vi "Check Protection.vi"(8 "error in (no error)":errorcluster, 10 "String in":string, 11 "SMC Protection in":refnum<class "SMC Protection.lvclass">) -> (0 "error out":errorcluster, 1 "Protection Error":errorcluster, 2 "String out":string, 3 "SMC Protection out":refnum<class "SMC Protection.lvclass">)   [LabVIEW 2021, in "Protections.lvlib" / "SMC Protection.lvclass"]
uses:
  SMC Protection.lvclass
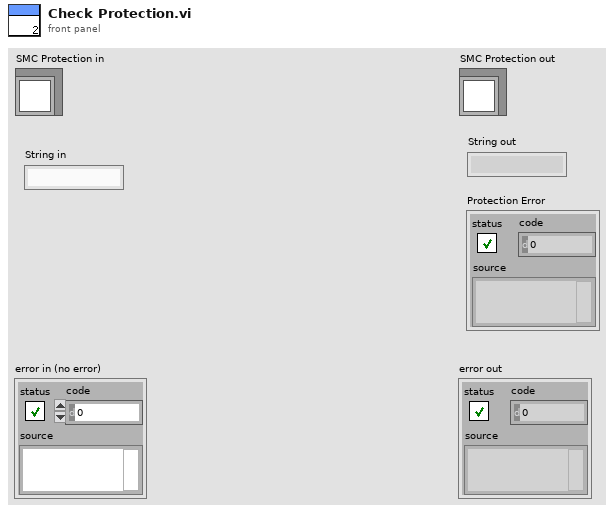
[diagram p1: front panel]
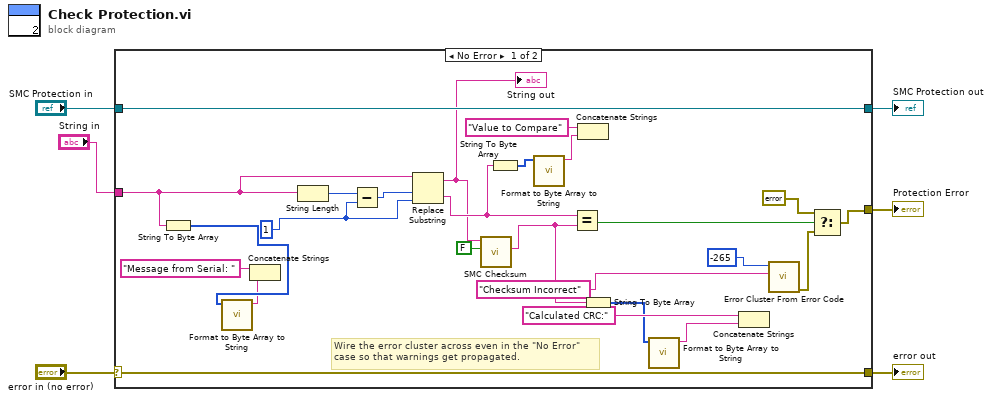
[diagram p0: block diagram]
diagram:
  n1 = case shown="No Error" "error in (no error)" {
    selector: "error in (no error)" -> [w30 w33]
    tunnel: [w30 w33] -> w5
    tunnel: [w31 w32] -> w3
    tunnel: "SMC Protection in" -> [w31 w32]
    tunnel: "String in" -> [w16 _]
    tunnel: [w21 _] -> w1
    frame No Error {
      w27 = 1
      # "Wire the error cluster across even in the \"No Error\"\ncase so that warnings get propagated."
      n2 = String To Byte Array(string=w16) -> (unsigned byte array=w15:u8[])
      n3 = call "Format to Byte Array to String.vi"("unsigned byte array"=w15) -> ("String"=w14:string)  [unwired: 10 in]
      n4 = Concatenate Strings("Message from Serial: " ("string"), w14) -> ()  [unwired: 1 out]
      n5 = String Length(string=w16) -> (length=w29:i32)
      n6 = Subtract(x=w29, y=w27) -> (x-y=w28:i32)
      n7 = Replace Substring(2:w27, 3:w28, 5:w16) -> (0:w12:string, 1:w7:string)  [unwired: 1 in]
      "String out" <- w7
      n8 = call "SMC Checksum.vi"("Pad"=FALSE, "String in"=w7) -> ("Checksum String"=w10:string)  [unwired: 8 in, 1 out]
      n9 = String To Byte Array(string=w12) -> (unsigned byte array=w13:u8[])
      n10 = call "Format to Byte Array to String.vi"("unsigned byte array"=w13) -> ("String"=w8:string)  [unwired: 10 in]
      n11 = Equal?(x=w12, y=w10) -> (x = y?=w24:bool)
      n12 = Concatenate Strings("Value to Compare" ("string"), w8) -> ()  [unwired: 1 out]
      n13 = String To Byte Array(string=w10) -> (unsigned byte array=w9:u8[])
      n14 = call "Format to Byte Array to String.vi"("unsigned byte array"=w9) -> ("String"=w11:string)  [unwired: 10 in]
      n15 = Concatenate Strings("Calculated CRC:" ("string"), w11) -> ()  [unwired: 1 out]
      n16 = call <vilib>:"Error Cluster From Error Code.vi"("error message (\"\")"="Checksum Incorrect" ("error message (\"\")"), "error code (0)"=-265) -> ("error out"=w23:errorcluster)  [unwired: 7 in]
      n17 = Select(t=errorcluster {"status"=FALSE, "code"=0, "source"=""}, s=w24, f=w23) -> (s? t:f=w21:errorcluster)
    }
    frame Error {
    }
  }
  "error out" <- w5
  "SMC Protection out" <- w3
  "Protection Error" <- w1
